vi "CAN_Write_Read64_2.vi"(7 "CAN frame":T1 {"payload" format="%x"; "timestamp" format="%<%.7X\n%x>T"; "type" items=["CAN Data"=0, "CAN Remote"=1, "CAN Bus Error"=2, "CAN 2.0 Data"=8, "CAN FD Data"=16, "CAN FD+BRS Data"=24, "J1939 Data"=192, "Delay"=224, "Log Trigger"=225, "Start Trigger"=226]; "identifier" format="%x"}, 8 "Error In":errorcluster, 9 "Numeric Request":u32, 10 "Write In":refnum<k21>, 11 "Read In":refnum<k21>) -> (0 "cluster":T3 {"data[0]"."payload" format="%x"; "data[0]"."timestamp" format="%<%.7X\n%x>T"; "data[0]"."type" items=["CAN Data"=0, "CAN Remote"=1, "CAN Bus Error"=2, "CAN 2.0 Data"=8, "CAN FD Data"=16, "CAN FD+BRS Data"=24, "J1939 Data"=192, "Delay"=224, "Log Trigger"=225, "Start Trigger"=226]; "data[0]"."identifier" format="%x"; "data[1]"."payload" format="%x"; "data[1]"."timestamp" format="%<%.7X\n%x>T"; "data[1]"."type" items=["CAN Data"=0, "CAN Remote"=1, "CAN Bus Error"=2, "CAN 2.0 Data"=8, "CAN FD Data"=16, "CAN FD+BRS Data"=24, "J1939 Data"=192, "Delay"=224, "Log Trigger"=225, "Start Trigger"=226]; "data[1]"."identifier" format="%x"; "data[2]"."payload" format="%x"; "data[2]"."timestamp" format="%<%.7X\n%x>T"; "data[2]"."type" items=["CAN Data"=0, "CAN Remote"=1, "CAN Bus Error"=2, "CAN 2.0 Data"=8, "CAN FD Data"=16, "CAN FD+BRS Data"=24, "J1939 Data"=192, "Delay"=224, "Log Trigger"=225, "Start Trigger"=226]; "data[2]"."identifier" format="%x"; "data[3]"."payload" format="%x"; "data[3]"."timestamp" format="%<%.7X\n%x>T"; "data[3]"."type" items=["CAN Data"=0, "CAN Remote"=1, "CAN Bus Error"=2, "CAN 2.0 Data"=8, "CAN FD Data"=16, "CAN FD+BRS Data"=24, "J1939 Data"=192, "Delay"=224, "Log Trigger"=225, "Start Trigger"=226]; "data[3]"."identifier" format="%x"; "data[4]"."payload" format="%x"; "data[4]"."timestamp" format="%<%.7X\n%x>T"; "data[4]"."type" items=["CAN Data"=0, "CAN Remote"=1, "CAN Bus Error"=2, "CAN 2.0 Data"=8, "CAN FD Data"=16, "CAN FD+BRS Data"=24, "J1939 Data"=192, "Delay"=224, "Log Trigger"=225, "Start Trigger"=226]; "data[4]"."identifier" format="%x"; "data[5]"."payload" format="%x"; "data[5]"."timestamp" format="%<%.7X\n%x>T"; "data[5]"."type" items=["CAN Data"=0, "CAN Remote"=1, "CAN Bus Error"=2, "CAN 2.0 Data"=8, "CAN FD Data"=16, "CAN FD+BRS Data"=24, "J1939 Data"=192, "Delay"=224, "Log Trigger"=225, "Start Trigger"=226]; "data[5]"."identifier" format="%x"; "data[6]"."payload" format="%x"; "data[6]"."timestamp" format="%<%.7X\n%x>T"; "data[6]"."type" items=["CAN Data"=0, "CAN Remote"=1, "CAN Bus Error"=2, "CAN 2.0 Data"=8, "CAN FD Data"=16, "CAN FD+BRS Data"=24, "J1939 Data"=192, "Delay"=224, "Log Trigger"=225, "Start Trigger"=226]; "data[6]"."identifier" format="%x"; "data[7]"."payload" format="%x"; "data[7]"."timestamp" format="%<%.7X\n%x>T"; "data[7]"."type" items=["CAN Data"=0, "CAN Remote"=1, "CAN Bus Error"=2, "CAN 2.0 Data"=8, "CAN FD Data"=16, "CAN FD+BRS Data"=24, "J1939 Data"=192, "Delay"=224, "Log Trigger"=225, "Start Trigger"=226]; "data[7]"."identifier" format="%x"; "data[8]"."payload" format="%x"; "data[8]"."timestamp" format="%<%.7X\n%x>T"; "data[8]"."type" items=["CAN Data"=0, "CAN Remote"=1, "CAN Bus Error"=2, "CAN 2.0 Data"=8, "CAN FD Data"=16, "CAN FD+BRS Data"=24, "J1939 Data"=192, "Delay"=224, "Log Trigger"=225, "Start Trigger"=226]; "data[8]"."identifier" format="%x"}, 1 "Error Out":errorcluster, 2 "Read Out":refnum<k21>, 3 "Write Out":refnum<k21>)   [LabVIEW 2023]
uses:
  <vilib>/xnet/xnet.llb/XNET Frame CAN.ctl
  <vilib>/xnet/xnet.llb/XNET Frame Type CAN.ctl
panel:
  out "ID Correct?":bool
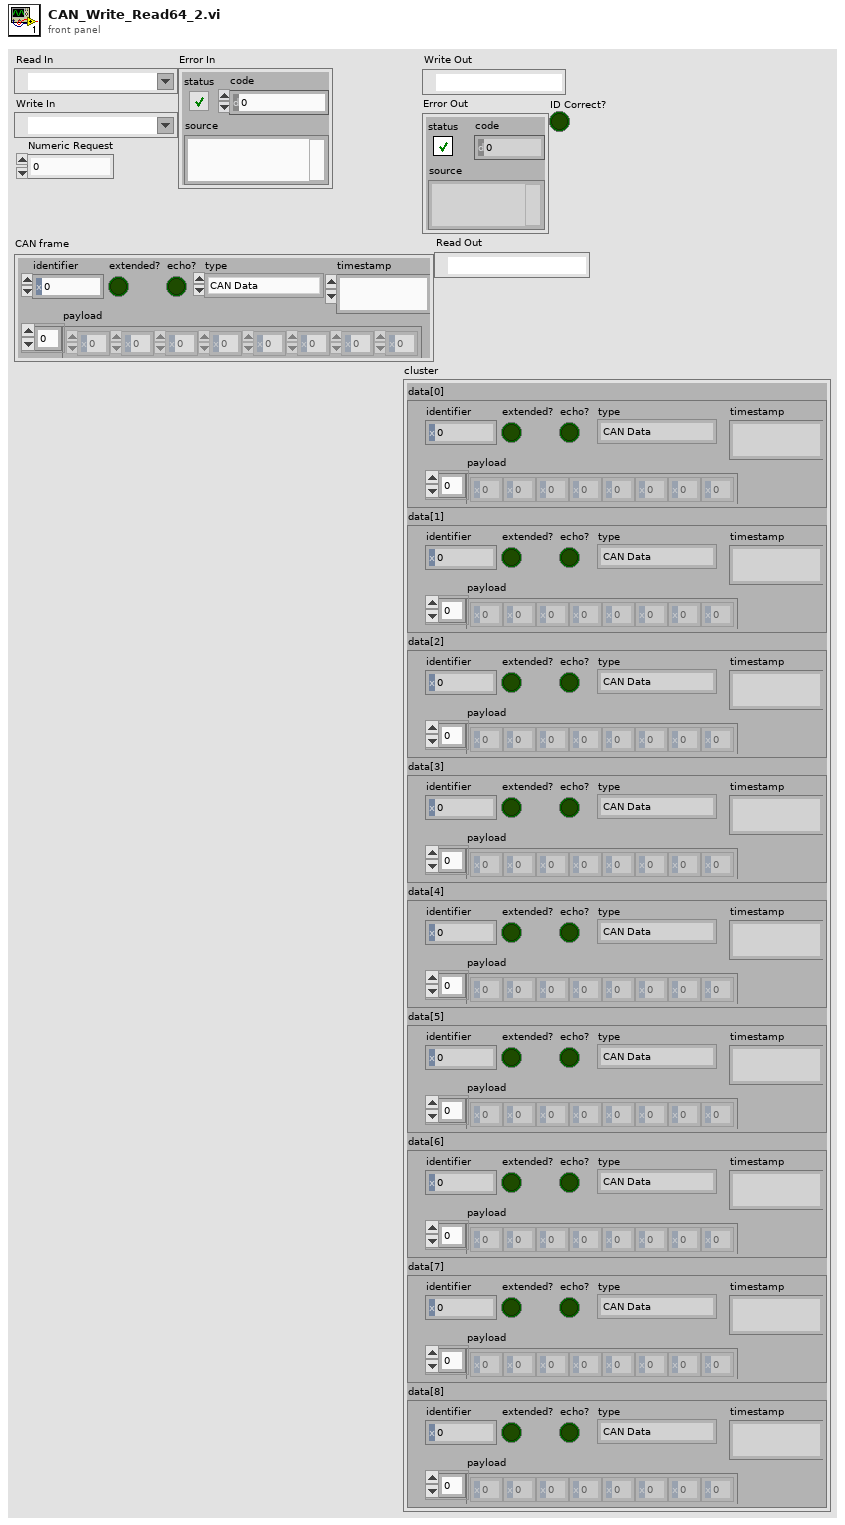
[diagram p1: front panel]
types:
  T1 = typedef "XNET Frame CAN.ctl" = cluster{"timestamp":timestamp, "payload":u8[], "identifier":u32, "type":T2, "extended?":bool, "echo?":bool}
  T2 = typedef "XNET Frame Type CAN.ctl" = u8
  T3 = cluster{"data[0]":T1, "data[1]":T1, "data[2]":T1, "data[3]":T1, "data[4]":T1, "data[5]":T1, "data[6]":T1, "data[7]":T1, "data[8]":T1}
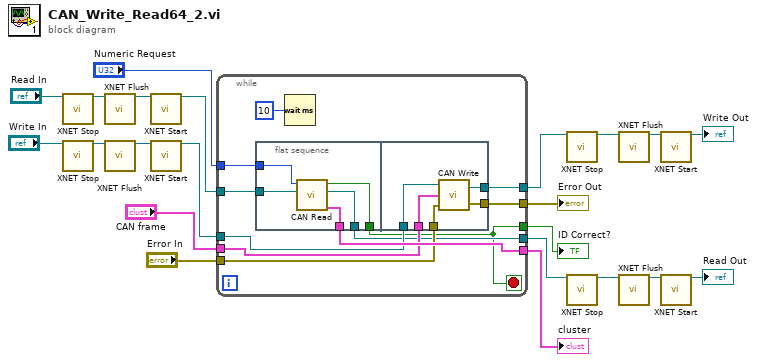
[diagram p0: block diagram]
diagram:
  n1 = call <vilib>:"XNET Stop.vi"("session in"="Read In") -> ("session out"=w16:refnum<k21>)  [unwired: 13 in, 1 out]
  n2 = call <vilib>:"XNET Stop.vi"("session in"="Write In") -> ("session out"=w18:refnum<k21>)  [unwired: 13 in, 1 out]
  n3 = call <vilib>:"XNET Flush.vi"("session in"=w16) -> ("session out"=w15:refnum<k21>)  [unwired: 13 in, 1 out]
  n4 = call <vilib>:"XNET Flush.vi"("session in"=w18) -> ("session out"=w17:refnum<k21>)  [unwired: 13 in, 1 out]
  n5 = call <vilib>:"XNET Start.vi"("session in"=w15) -> ("session out"=w13:refnum<k21>)  [unwired: 13 in, 1 out]
  n6 = call <vilib>:"XNET Start.vi"("session in"=w17) -> ("session out"=w20:refnum<k21>)  [unwired: 13 in, 1 out]
  n7 = while {
    tunnel: w13 -> [w31]
    tunnel: [w25] -> w5
    tunnel: "Error In" -> [w29]
    tunnel: w20 -> [w27]
    tunnel: "CAN frame" -> [w28]
    tunnel: [w26] -> w12
    tunnel: "Numeric Request" -> [w32]
    tunnel: [w30] -> w10
    tunnel: [w24] -> w9
    tunnel: [w23] -> w1
    stop <- w23 stop-if-true
    n8 = flat-sequence {
      tunnel: w32 -> [w37]
      tunnel: w31 -> [w38]
      tunnel: [w34] -> w30
      tunnel: [w35] -> w24
      tunnel: [w36] -> w23
      tunnel: w29 -> [w43]
      tunnel: w28 -> [w42]
      tunnel: w27 -> [w41]
      tunnel: [w40] -> w26
      tunnel: [w39] -> w25
      frame #0 {
        n9 = call "CAN Read.vi"("Read In"=w38, "Numeric Request"=w37) -> ("cluster"=w34:T3, "Read Out"=w35:refnum<k21>, "ID Correct?"=w36:bool)  [unwired: 2 in, 1 out]
      }
      frame #1 {
        n10 = call "CAN Write.vi"("Error In"=w43, "CAN frame"=w42, "Write In"=w41) -> ("Error Out"=w40:errorcluster, "Write Out"=w39:refnum<k21>)
      }
    }
    n11 = Wait (ms)(milliseconds to wait=u32 10) -> ()  [unwired: 1 out]
  }
  "Error Out" <- w12
  "ID Correct?" <- w1
  "cluster" <- w10
  n12 = call <vilib>:"XNET Stop.vi"("session in"=w5) -> ("session out"=w4:refnum<k21>)  [unwired: 13 in, 1 out]
  n13 = call <vilib>:"XNET Stop.vi"("session in"=w9) -> ("session out"=w8:refnum<k21>)  [unwired: 13 in, 1 out]
  n14 = call <vilib>:"XNET Flush.vi"("session in"=w4) -> ("session out"=w3:refnum<k21>)  [unwired: 13 in, 1 out]
  n15 = call <vilib>:"XNET Flush.vi"("session in"=w8) -> ("session out"=w7:refnum<k21>)  [unwired: 13 in, 1 out]
  n16 = call <vilib>:"XNET Start.vi"("session in"=w3) -> ("session out"=→"Write Out":refnum<k21>)  [unwired: 13 in, 1 out]
  n17 = call <vilib>:"XNET Start.vi"("session in"=w7) -> ("session out"=→"Read Out":refnum<k21>)  [unwired: 13 in, 1 out]
